vi "get vi details.vi"(8 "error in (no error)":errorcluster, 11 "path":string) -> (0 "error out":errorcluster, 2 "vi_blockdiagram":picture, 3 "vi_description":string)   [LabVIEW 2020]
doc: "Takes a VI path (.vi files). Returns the description and screenshot of block diagram. Use this to understand what VI is doing."
uses:
  G-AI Core/G-AI Core.lvlib
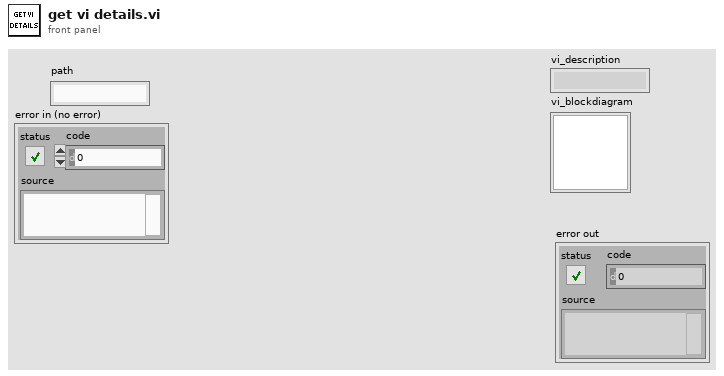
[diagram p1: front panel]
types:
  T1 = typedef "imagedata.ctl" = cluster{"image type":i32, "image depth":i32, "image":u8[], "mask":u8[], "colors":u32[], "Rectangle":cluster{"left":i16, "top":i16, "right":i16, "bottom":i16}}
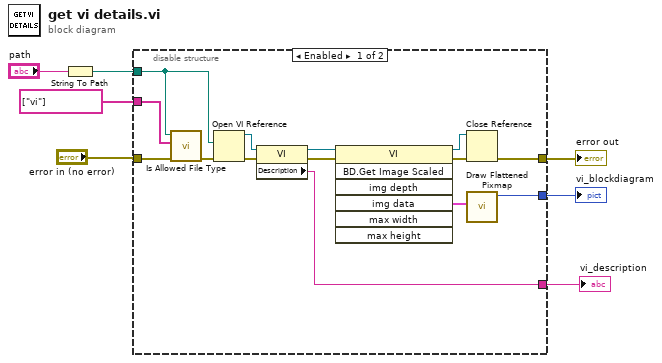
[diagram p0: block diagram]
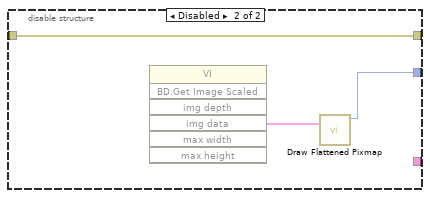
[diagram p2: hidden frame]
diagram:
  n1 = String To Path(string="path") -> (path=w3:path)
  n2 = disable-structure shown="Enabled" {
    disable-tunnel: [w19 _] -> w6
    disable-tunnel: [w15 w22] -> w5
    disable-tunnel: [w12 w24] -> w4
    disable-tunnel: "error in (no error)" -> [w11 w24]
    disable-tunnel: w3 -> [w10 _]
    disable-tunnel: string[] ["vi"] ("y") -> [w9 _]
    frame Enabled {
      n3 = call "Is Allowed File Type.vi"("error in (no error)"=w11, "y"=w9, "Path"=w10) -> ("error out"=w8:errorcluster)  [unwired: 8 in]
      n4 = Open VI Reference(vi path=w10, error in (no error)=w8) -> (vi reference=w20:refnum<vi>, error out=w21:errorcluster)  [unwired: 4 in]
      n5 = property class="VI"(reference=w20, error in=w21) -> (reference out=w16:refnum<vi>, error out=w17:errorcluster, "Description"=w19:string)
      n6 = invoke class="VI" method="BD.Get Image Scaled"(reference=w16, error in=w17) -> (reference out=w13:refnum<vi>, error out=w14:errorcluster, "img data"=w18:T1)  [unwired: 5 in, 4 out]
      n7 = Close Reference(reference=w13, error in (no error)=w14) -> (error out=w12:errorcluster)
      n8 = call <vilib>:"Draw Flattened Pixmap.vi"("image data"=w18) -> ("new picture"=w15:picture)  [unwired: 8 in]
    }
    frame Disabled {
      n9 = invoke class="VI" method="BD.Get Image Scaled"() -> ("img data"=w23:T1)  [unwired: 7 in, 6 out]
      n10 = call <vilib>:"Draw Flattened Pixmap.vi"("image data"=w23) -> ("new picture"=w22:picture)  [unwired: 8 in]
    }
  }
  "vi_description" <- w6
  "vi_blockdiagram" <- w5
  "error out" <- w4
